vi "Compare Strings.vi"(5 "ignore case? (T)":bool=TRUE, 9 "String2":string, 10 "String1":string) -> (2 "Match":bool)   [LabVIEW 2012]
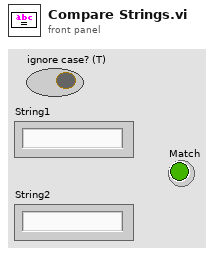
[diagram p1: front panel]
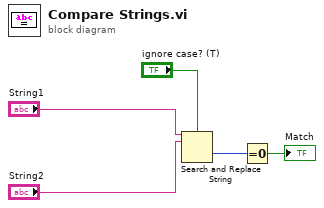
[diagram p0: block diagram]
diagram:
  n1 = Search and Replace String(case sensitive?="ignore case? (T)", input string="String1", search string="String2") -> (offset past replacement=w2:i32)  [unwired: 5 in, 3 out]
  n2 = Equal To 0?(x=w2) -> (x = 0?=→"Match":bool)
